vi "Export - Strip Controller Path.vi"(8 "error in (no error)":errorcluster, 10 "Channel Path":string, 11 "Controller Path":string) -> (0 "error out":errorcluster, 2 "Stripped Path":string)   [LabVIEW 2016, in "UDP-Custom-Device System Explorer.lvlib"]
uses:
  UDP-Custom-Device System Explorer.lvlib
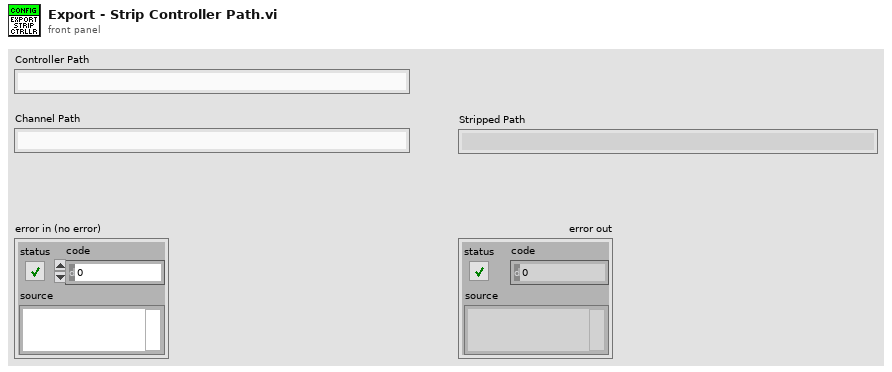
[diagram p1: front panel]
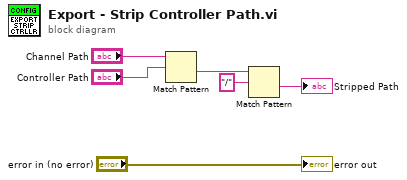
[diagram p0: block diagram]
diagram:
  n1 = Match Pattern(string="Channel Path", regular expression="Controller Path") -> (after substring=w2:string)  [unwired: 1 in, 3 out]
  n2 = Match Pattern(string=w2, regular expression="/") -> (after substring=→"Stripped Path":string)  [unwired: 1 in, 3 out]
  "error out" <- "error in (no error)"
